vi "prime_odd_even_composite_for_n.vi"() -> ()   [LabVIEW 2019]
panel:
  in  "?":bool
  out "COMPOSITE NUMBERS":i32[](array[numeric])
  out "ODD NUMBERS":i32[](array[numeric])
  out "EVEN NUMBERS":i32[](array[numeric])
  out "PRIME NUMBERS":i32[](array[numeric])
  in  "ENTER THE NUMBER":i32
  # "num_type finder"
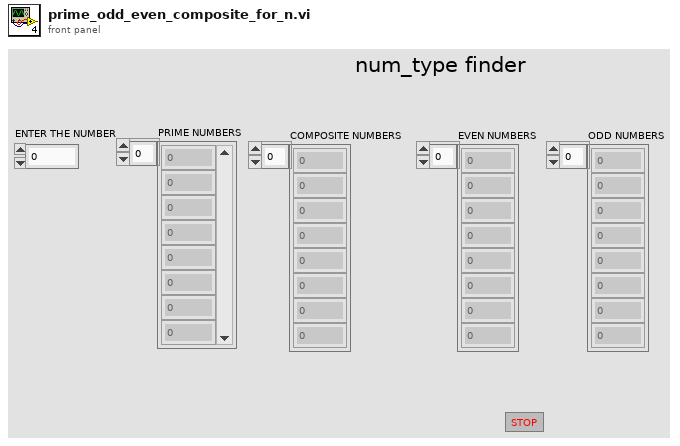
[diagram p1: front panel]
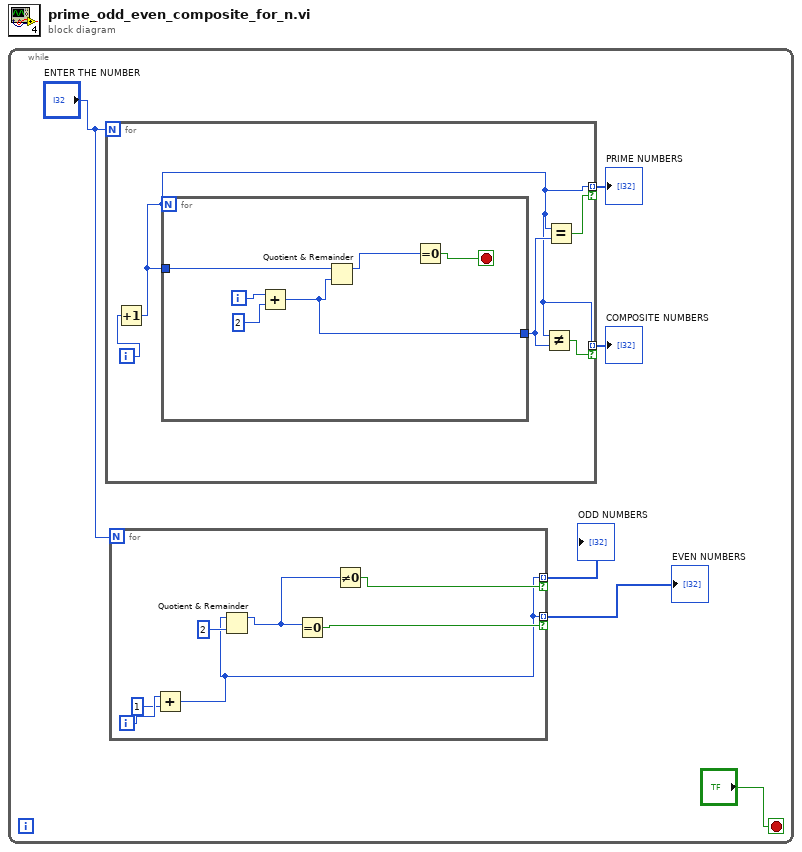
[diagram p0: block diagram]
diagram:
  n1 = while {
    stop <- "?" stop-if-true
    n2 = for {
      N: "ENTER THE NUMBER" -> [_]
      tunnel: [w14] -> w6 mode=indexing if=w18
      tunnel: [w14] -> w2 mode=indexing if=w16
      i -> [w15]
      n3 = Increment(x=w15) -> (x+1=w14:i32)
      n4 = for {
        N: w14 -> [_]
        tunnel: w14 -> [w22]
        tunnel: [w19] -> w17
        i -> [w24]
        stop <- w20 stop-if-true
        n5 = Add(x=w24, y=2 ("x")) -> (x+y=w19:i32)
        n6 = Quotient & Remainder(x=w22, y=w19) -> (x-y*floor(x/y)=w21:i32)  [unwired: 1 out]
        n7 = Equal To 0?(x=w21) -> (x = 0?=w20:bool)
      }
      n8 = Not Equal?(x=w14, y=w17) -> (x != y?=w16:bool)
      n9 = Equal?(x=w14, y=w17) -> (x = y?=w18:bool)
    }
    "PRIME NUMBERS" <- w6
    "COMPOSITE NUMBERS" <- w2
    n10 = for {
      N: "ENTER THE NUMBER" -> [_]
      tunnel: [w7] -> w4 mode=indexing if=w12
      tunnel: [w7] -> w3 mode=indexing if=w10
      i -> [w9]
      n11 = Add(x=w9, y=1) -> (x+y=w7:i32)
      n12 = Quotient & Remainder(x=w7, y=2) -> (x-y*floor(x/y)=w11:i32)  [unwired: 1 out]
      n13 = Equal To 0?(x=w11) -> (x = 0?=w12:bool)
      n14 = Not Equal To 0?(x=w11) -> (x != 0?=w10:bool)
    }
    "EVEN NUMBERS" <- w4
    "ODD NUMBERS" <- w3
  }
